vi "HEWH Get Last Draw Timestamp.vi"(6 "Use Specific Time":bool, 7 "Search Software Elapsed Time":dbl, 8 "error in (no error)":errorcluster, 9 "FHD-After 1 hour":dbl[][](array[numeric]), 10 "Test Data-Start to End DBL":dbl[][](array[numeric]), 11 "Softw Elapsed Time\n Full Data Set (Each Draw)":dbl[][](array[numeric])) -> (0 "error out":errorcluster, 2 "Elapsed Time - Last Draw Timestamp":dbl, 3 "Software Elapsed Timestamp of Last Draw":dbl)   [LabVIEW 2023]
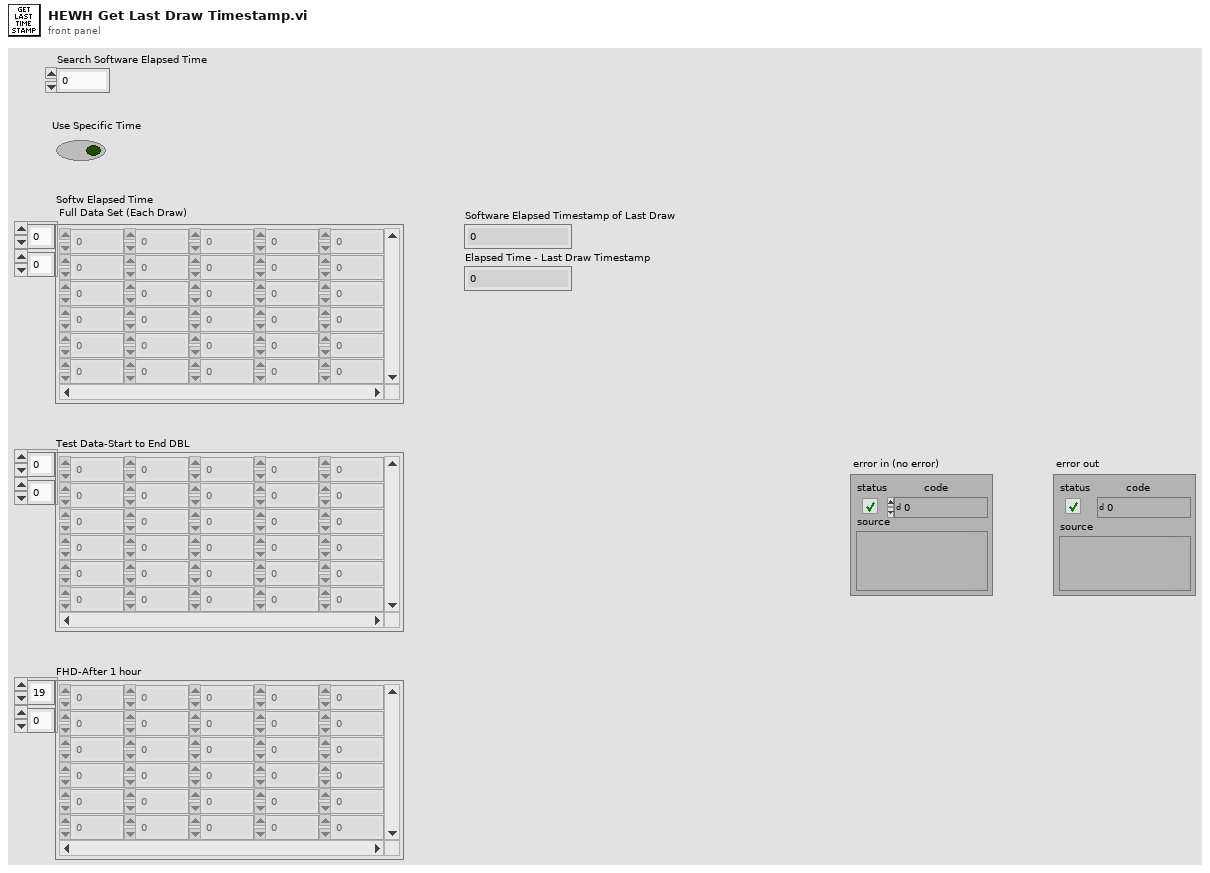
[diagram p1: front panel]
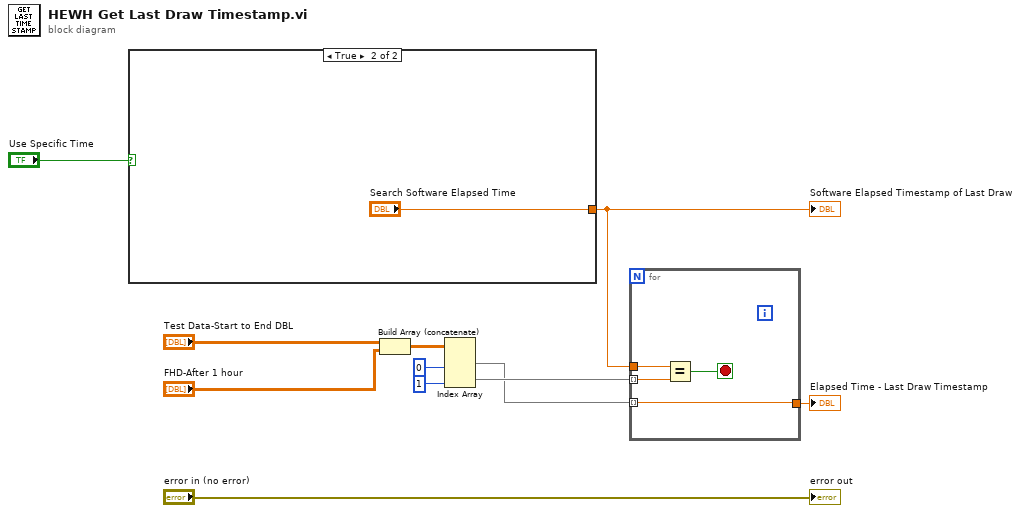
[diagram p0: block diagram]
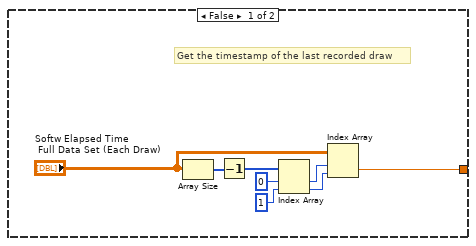
[diagram p2: hidden frame]
diagram:
  n1 = case shown="True" "Use Specific Time" {
    tunnel: [w19 "Search Software Elapsed Time"] -> w4
    frame False {
      # "Get the timestamp of the last recorded draw"
      n2 = Array Size(array="Softw Elapsed Time\n Full Data Set (Each Draw)") -> (size(s)=w12:i32[])
      n3 = Decrement(x=w12) -> (x-1=w13:i32[])
      n4 = Index Array(array=w13, index #1=0 ("index"), index #2=1 ("index")) -> (element #1=w17:i32, element #2=w18:i32)
      n5 = Index Array(array="Softw Elapsed Time\n Full Data Set (Each Draw)", index (row)=w17, index (col)=w18) -> (element=w19:dbl)
    }
    frame True {
    }
  }
  "Software Elapsed Timestamp of Last Draw" <- w4
  n6 = Build Array (concatenate)("Test Data-Start to End DBL", "FHD-After 1 hour") -> (w8:dbl[][])
  n7 = Index Array(array=w8, index (col) #1=0 ("index (row)"), index (col) #2=1 ("disabled index (col)")) -> (element #1=w3:dbl[], element #2=w5:dbl[])  [unwired: 2 in]
  n8 = for {
    tunnel: w5 -> [w24] mode=indexing
    tunnel: w4 -> [w23]
    tunnel: w3 -> [w21] mode=indexing
    tunnel: [w21] -> w2
    stop <- w22 stop-if-true
    n9 = Equal?(x=w23, y=w24) -> (x = y?=w22:bool)
  }
  "Elapsed Time - Last Draw Timestamp" <- w2
  "error out" <- "error in (no error)"
